vi "Test.vi"() -> ()   [LabVIEW 2018]
uses:
  <vilib>/picture/picture.llb/imagedata.ctl
  <userlib>/_OpenG.lib/numeric/numeric.llb/Random Number Within Range - I32__ogtk.vi
panel:
  out "out":picture
  out "origin":picture
  in  "path to PNG file":path=path "D:/LabVIEW Work/Pets/Waterfall/pops.png"
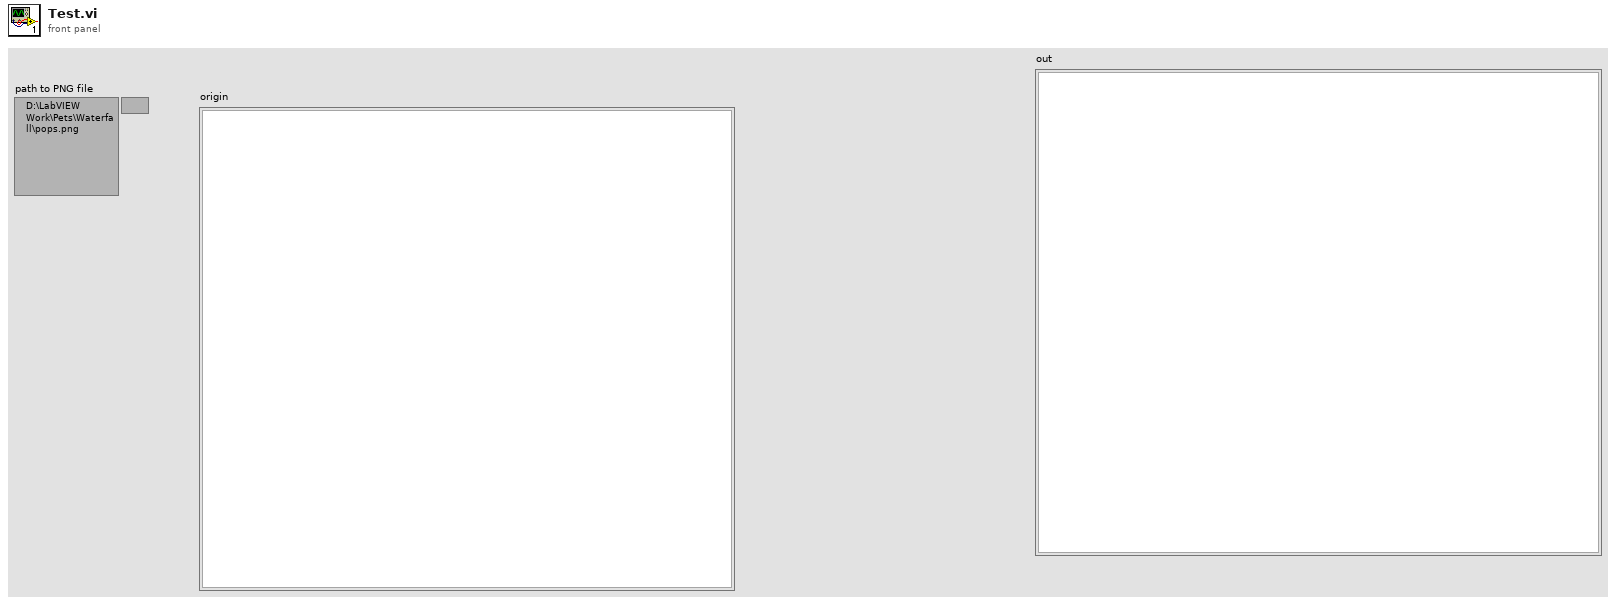
[diagram p1: front panel]
types:
  T1 = typedef "imagedata.ctl" = cluster{"image type":i32, "image depth":i32, "image":u8[], "mask":u8[], "colors":u32[], "Rectangle":cluster{"left":i16, "top":i16, "right":i16, "bottom":i16}}
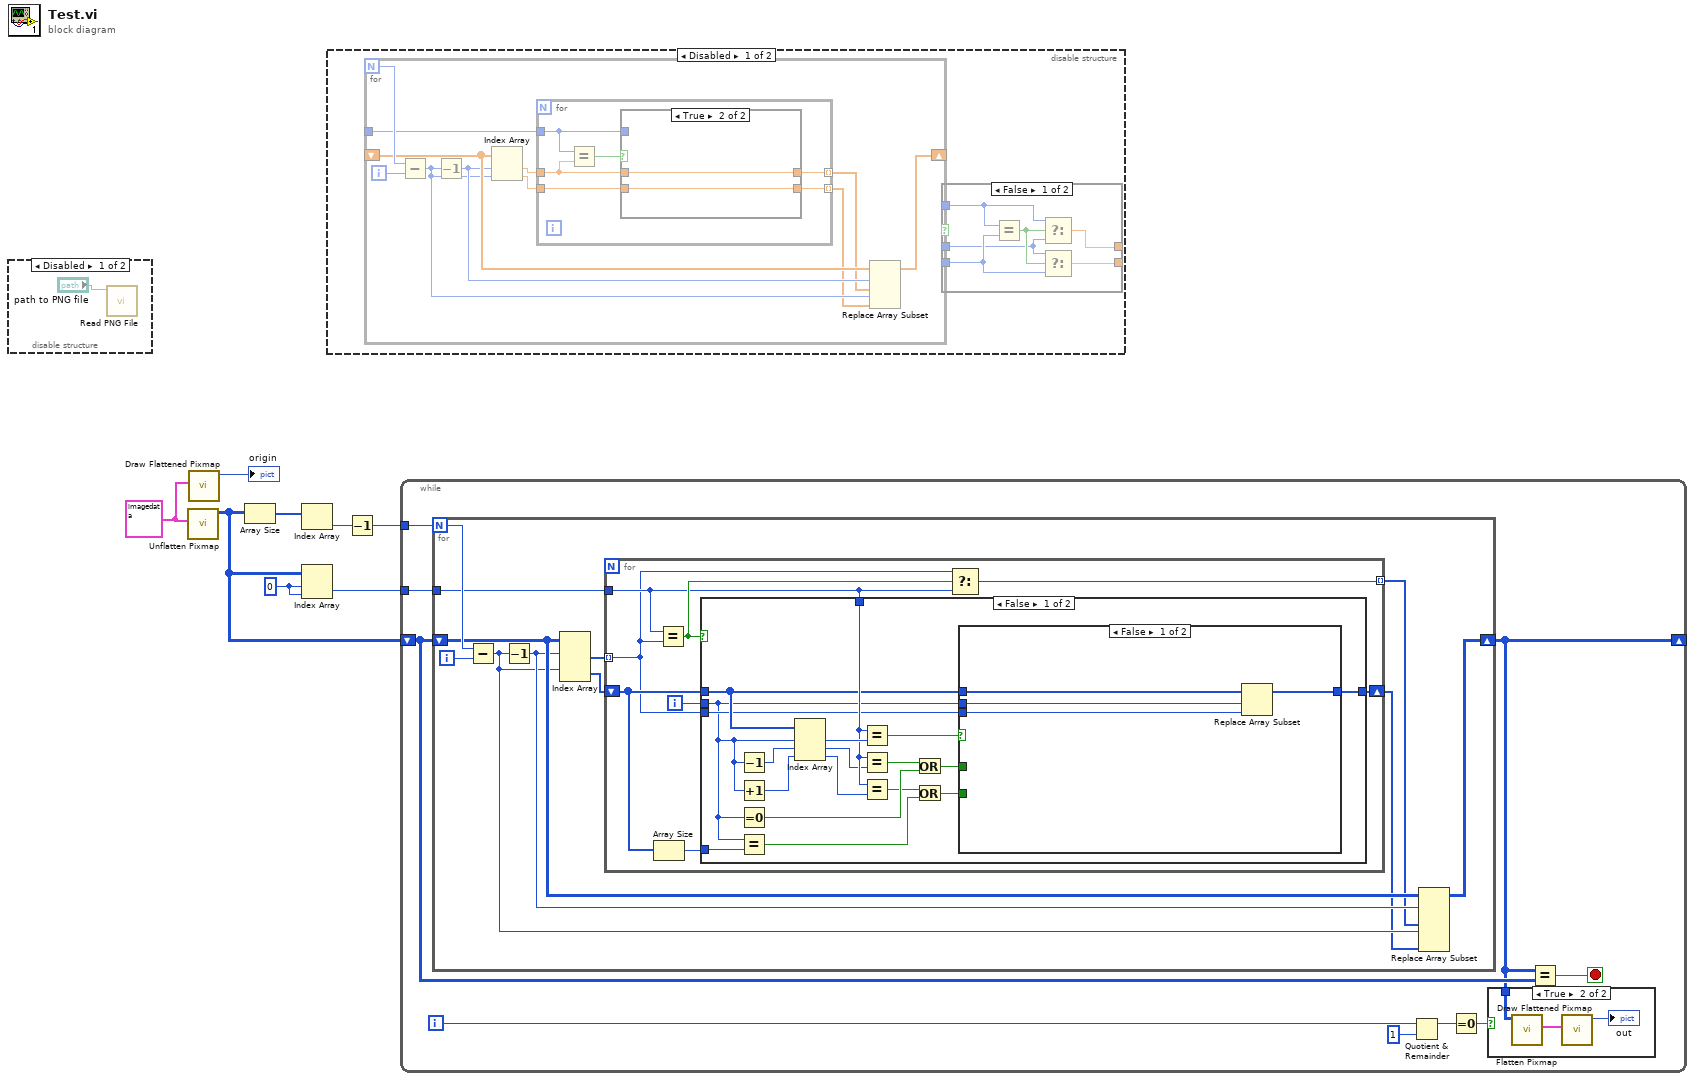
[diagram p0: block diagram]
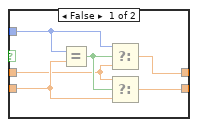
[diagram p3: hidden frame]
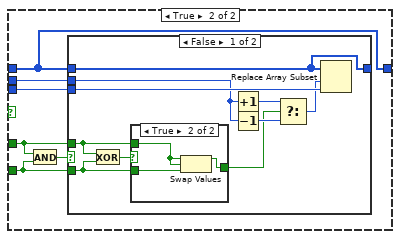
[diagram p7: hidden frame]
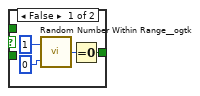
[diagram p8: hidden frame]
diagram:
  w2 = T1 {"image type"=0, "image depth"=24, "image"=array[740862 elements], "mask"=[], "colors"=[], "Rectangle"={"left"=0, "top"=0, "right"=521, "bottom"=474}} ("image data")
  w7 = 0 ("index (row)")
  n1 = disable-structure shown="Disabled" {
    frame Disabled {
      n2 = call <vilib>:"Read PNG File.vi"("path to PNG file"="path to PNG file") -> ()  [unwired: 8 in, 3 out]
    }
    frame Enabled {
    }
  }
  n3 = call <vilib>:"Unflatten Pixmap.vi"("image data"=w2) -> ("24-bit pixmap"=w1:u32[][])  [unwired: 4 in, 6 out]
  n4 = call <vilib>:"Draw Flattened Pixmap.vi"("image data"=w2) -> ("new picture"=→"origin":picture)  [unwired: 8 in]
  n5 = Array Size(array=w1) -> (size(s)=w6:i32[])
  n6 = Index Array(array=w6) -> (element=w5:i32)  [unwired: 1 in]
  n7 = Index Array(array=w1, index (row)=w7, index (col)=w7) -> (element=w3:u32)
  n8 = disable-structure shown="Disabled" {
    frame Disabled {
      n9 = for {
        N -> [w28]
        tunnel: _ -> [w24]
        shift-right: [w18] -> _
        shift-left: _ -> [w23]
        i -> [w27]
        n10 = Subtract(x=w28, y=w27) -> (x-y=w20:i32)
        n11 = Decrement(x=w20) -> (x-1=w22:i32)
        n12 = Index Array(array=w23, index #1=w22, index #2=w20) -> (element #1=w26:dbl, element #2=w25:dbl)
        n13 = for {
          tunnel: w26 -> [w32]
          tunnel: w24 -> [w29]
          tunnel: w25 -> [w33]
          tunnel: [w31] -> w21 mode=indexing
          tunnel: [w30] -> w19 mode=indexing
          n14 = Equal?(x=w29, y=w32) -> (x = y?=w34:bool)
          n15 = case shown="True" w34 {
            tunnel: w33 -> [w40 w41]
            tunnel: w32 -> [w35 w42]
            tunnel: [w38 w42] -> w31
            tunnel: [w39 w41] -> w30
            tunnel: w29 -> [w36 _]
            frame False {
              n16 = Equal?(x=w36, y=w40) -> (x = y?=w37:bool)
              n17 = Select(t=w36, s=w37, f=w35) -> (s? t:f=w38:dbl)
              n18 = Select(t=w35, s=w37, f=w40) -> (s? t:f=w39:dbl)
            }
            frame True {
            }
          }
        }
        n19 = Replace Array Subset(array=w23, new element #1=w21, index #1=w22, new element #2=w19, index #2=w20) -> (w18:dbl[])
      }
      n20 = case shown="False" {
        selector: _ -> [_ _]
        tunnel: _ -> [w15 w16]
        tunnel: _ -> [w10 w17]
        tunnel: [w13 w17] -> _
        tunnel: [w14 w16] -> _
        tunnel: _ -> [w11 _]
        frame False {
          n21 = Equal?(x=w11, y=w15) -> (x = y?=w12:bool)
          n22 = Select(t=w11, s=w12, f=w10) -> (s? t:f=w13:dbl)
          n23 = Select(t=w10, s=w12, f=w15) -> (s? t:f=w14:dbl)
        }
        frame True {
        }
      }
    }
    frame Enabled {
    }
  }
  n24 = Decrement(x=w5) -> (x-1=w4:i32)
  n25 = while {
    tunnel: w4 -> [w51]
    tunnel: w3 -> [w50]
    shift-right: [w47] -> _
    shift-left: w1 -> [w49]
    i -> [w46]
    stop <- w48 stop-if-true
    n26 = for {
      N: w51 -> [w65]
      tunnel: w50 -> [w62]
      shift-right: [w56] -> w47
      shift-left: w49 -> [w61]
      i -> [w64]
      n27 = Subtract(x=w65, y=w64) -> (x-y=w58:i32)
      n28 = Decrement(x=w58) -> (x-1=w60:i32)
      n29 = Index Array(array=w61, index (row) #1=w60, index (row) #2=w58) -> (element #1=w63:u32[], element #2=w55:u32[])  [unwired: 2 in]
      n30 = for {
        tunnel: w63 -> [w66] mode=indexing
        tunnel: w62 -> [w70]
        tunnel: [w73] -> w59 mode=indexing
        shift-right: [w71] -> w57
        shift-left: w55 -> [w69]
        i -> [w68]
        n31 = Array Size(array=w69) -> (size(s)=w67:i32)
        n32 = Equal?(x=w70, y=w66) -> (x = y?=w72:bool)
        n33 = case shown="False" w72 {
          tunnel: w69 -> [w79 w120]
          tunnel: [w76 w120] -> w71
          tunnel: w68 -> [w77 _]
          tunnel: w70 -> [w87 _]
          tunnel: w67 -> [w90 _]
          tunnel: w66 -> [w78 _]
          frame False {
            n34 = Decrement(x=w77) -> (x-1=w89:i32)
            n35 = Increment(x=w77) -> (x+1=w88:i32)
            n36 = Equal To 0?(x=w77) -> (x = 0?=w83:bool)
            n37 = Equal?(x=w77, y=w90) -> (x = y?=w81:bool)
            n38 = Index Array(array=w79, index #1=w77, index #2=w89, index #3=w88) -> (element #1=w91:u32, element #2=w86:u32, element #3=w85:u32)
            n39 = Equal?(x=w87, y=w91) -> (x = y?=w80:bool)
            n40 = Equal?(x=w87, y=w86) -> (x = y?=w84:bool)
            n41 = Equal?(x=w87, y=w85) -> (x = y?=w82:bool)
            n42 = Or(x=w84, y=w83) -> (x .or. y?=w75:bool)
            n43 = Or(x=w82, y=w81) -> (x .or. y?=w74:bool)
            n44 = case shown="False" w80 {
              tunnel: w79 -> [w95 w96]
              tunnel: w78 -> [w94 w100]
              tunnel: w77 -> [w93 w99]
              tunnel: [w92 w96] -> w76
              tunnel: w75 -> [_ w98]
              tunnel: w74 -> [_ w97]
              frame False {
                n45 = Replace Array Subset(array=w95, new element=w94, index=w93) -> (w92:u32[])
              }
              frame True {
                n46 = And(x=w98, y=w97) -> (x .and. y?=w101:bool)
                n47 = case shown="False" w101 {
                  tunnel: w96 -> [w102 w119]
                  tunnel: [w102 w119] -> _
                  tunnel: w100 -> [w111 _]
                  tunnel: w99 -> [w108 _]
                  tunnel: w98 -> [w103 _]
                  tunnel: w97 -> [w104 _]
                  frame False {
                    n48 = Exclusive Or(1:w104, 2:w103) -> (0:w106:bool)
                    n49 = case shown="True" w106 {
                      tunnel: [w112 w116] -> w105
                      tunnel: w104 -> [_ w118]
                      tunnel: w103 -> [_ w117]
                      frame False {
                        n50 = call-poly <userlib>:"Random Number Within Range__ogtk.vi"("High"=1, "Low"=0) -> ("Random Number"=w113:i32)  [unwired: 3 in]
                        n51 = Equal To 0?(x=w113) -> (x = 0?=w112:bool)
                      }
                      frame True {
                        n52 = Swap Values(12:w117, 13:w117, 14:w118) -> (1:w116:bool)  [unwired: 1 out]
                      }
                    }
                    n53 = Increment(x=w108) -> (x+1=w109:i32)
                    n54 = Decrement(x=w108) -> (x-1=w107:i32)
                    n55 = Select(t=w109, s=w105, f=w107) -> (s? t:f=w110:i32)
                    n56 = Replace Array Subset(array=w102, new element=w111, index=w110) -> ()  [unwired: 1 out]
                  }
                  frame True {
                  }
                }
              }
            }
          }
          frame True {
            # "current pixel is empty\nthere is nothing to fall"
          }
        }
        n57 = Select(t=w66, s=w72, f=w70) -> (s? t:f=w73:u32)
      }
      n58 = Replace Array Subset(array=w61, new element #1=w59, index (row) #1=w60, new element #2=w57, index (row) #2=w58) -> (w56:u32[][])  [unwired: 2 in]
    }
    n59 = Quotient & Remainder(x=w46, y=1) -> (x-y*floor(x/y)=w43:i32)  [unwired: 1 out]
    n60 = Equal To 0?(x=w43) -> (x = 0?=w44:bool)
    n61 = case shown="True" w44 {
      tunnel: w47 -> [_ w52]
      frame False {
      }
      frame True {
        n62 = call <vilib>:"Flatten Pixmap.vi"("24-bit pixmap"=w52) -> ("image data"=w54:T1)  [unwired: 10 in]
        n63 = call <vilib>:"Draw Flattened Pixmap.vi"("image data"=w54) -> ("new picture"=→"out":picture)  [unwired: 8 in]
      }
    }
    n64 = Equal?(x=w47, y=w49) -> (x = y?=w48:bool)
  }
